vi "Connection Handler.vi"(6 "connection reference":refnum<data-value>, 8 "UUID":string, 9 "Data Model":refnum<class "Device Data Model.lvclass">, 11 "TCP slave":refnum<class "TCP Slave.lvclass">) -> ()   [LabVIEW 2021, in "TCP Slave.lvclass"]
doc: "Handles new connections by waiting on TCP requests. When data is received, it will execute the modbus data unit and write the return data back onto the bus. It handles one request at a time."
uses:
  TCP Slave.lvclass
  TCP Slave.lvclass/TCP Slave.ctl
  Handler State.ctl
  Transmission Data Unit/Transmission Data Unit.lvclass
  Data Model/Device Data Model.lvclass
  Network Slave.lvclass
  C:/my_projects/projects/Algorithms/Labview/21/Modbus_v121c/Network Protocol/Network Slave/Network Slave.lvclass
  C:/my_projects/projects/Algorithms/Labview/21/Modbus_v121c/Network Protocol/Network Protocol.lvclass
  C:/my_projects/projects/Algorithms/Labview/21/Modbus_v121c/Network Protocol/Network Slave/TCP/TCP Slave.lvclass
  Connection.ctl
panel:
  in  "stop":bool
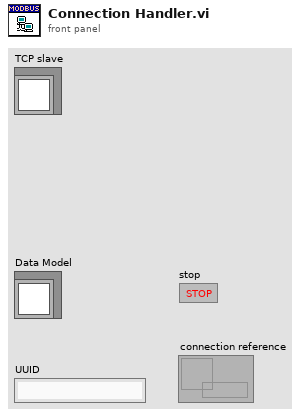
[diagram p1: front panel]
types:
  T1 = typedef "TCP Slave.lvclass/Handler State.ctl" = enum16{"Check Notifier", "Wait on Connection", "Quit"}
  T2 = typedef "TCP Slave.lvclass/Connection.ctl" = cluster{"Connected?":bool, "IP address":string, "connection error":errorcluster}
  T3 = typedef "TCP Slave.lvclass/Connection Counter.ctl" = cluster{"Currently Connected":u32, "Connection Records":refnum<data-value>[]}
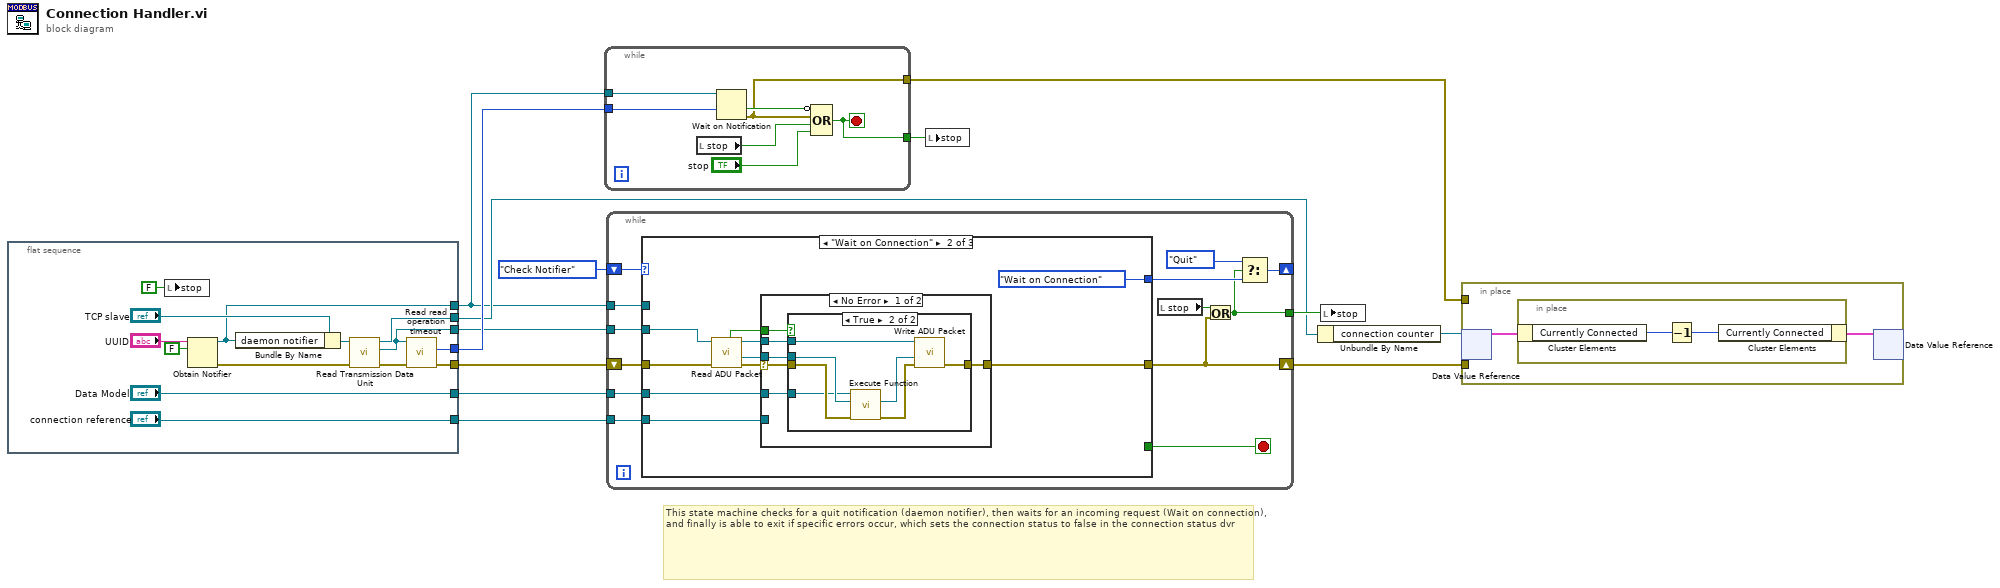
[diagram p0: block diagram]
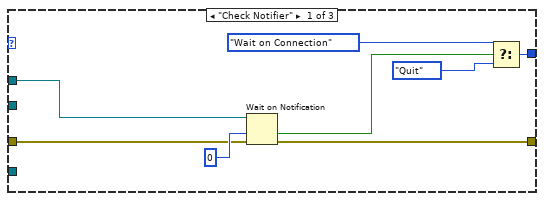
[diagram p2: hidden frame]
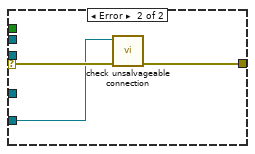
[diagram p4: hidden frame]
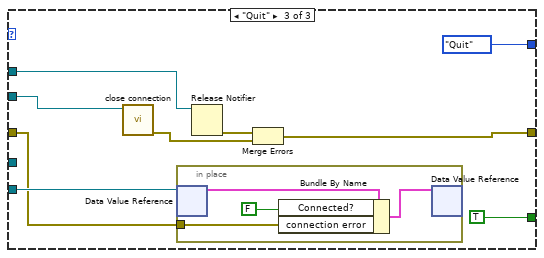
[diagram p5: hidden frame]
diagram:
  # "This state machine checks for a quit notification (daemon notifier), then waits for an incoming request (Wait on connection), and finally is able to exit if specific errors occur, which sets the connection status to false in the connection status dvr"
  n1 = flat-sequence {
    tunnel: ["connection reference"] -> w12
    tunnel: ["Data Model"] -> w11
    tunnel: [w20] -> w6
    tunnel: [w19] -> w5
    tunnel: [w17] -> w4
    tunnel: [w16] -> w1
    tunnel: [w14] -> w3
    frame #0 {
      n2 = local write "stop"(FALSE ("stop")) -> ()
      n3 = Obtain Notifier(name (unnamed)="UUID", notification data type=FALSE) -> (notifier out=w16:refnum<notifier>, error out=w21:errorcluster)  [unwired: 2 in, 1 out]
      n4 = Bundle By Name(cluster="TCP slave", "daemon notifier"=w16) -> (w18:refnum<class "TCP Slave.lvclass">)
      n5 = call "Read Transmission Data Unit.vi"("error in (no error)"=w21, "Network Slave in"=w18) -> ("error out"=w22:errorcluster, "Transmission Data Unit"=w14:refnum<class "Transmission Data Unit.lvclass">, "Network Slave out"=w17:refnum<class "TCP Slave.lvclass">)  [unwired: 7 in]
      n6 = call "Read read operation timeout.vi"("error in (no error)"=w22, "transmission data unit in"=w14) -> ("error out"=w20:errorcluster, "read operation timeout"=w19:i32)  [unwired: 7 in, 1 out]
    }
  }
  n7 = while {
    tunnel: w1 -> [w34]
    tunnel: [w31] -> w8
    tunnel: [w30] -> w2
    tunnel: w5 -> [w28]
    stop <- w31 stop-if-true
    n8 = local read "stop"() -> (w32:bool)
    n9 = Wait on Notification(notifier=w34, timeout in ms (-1)=w28) -> (timed out?=w33:bool, error out=w30:errorcluster)  [unwired: 2 in, 2 out]
    n10 = Compound Arithmetic op=OR(invert w33, w30, w32, "stop") -> (w31:bool)
  }
  n11 = while {
    shift-right: [w45] -> _
    shift-left: Handler_State."Check Notifier" ("Listener State") -> [w47]
    shift-right: [w37] -> w10
    shift-left: w6 -> [w42]
    tunnel: w12 -> [w40]
    tunnel: w11 -> [w39]
    tunnel: [w36] -> w7
    tunnel: w1 -> [w41]
    tunnel: w3 -> [w35]
    stop <- w43 stop-if-true
    n12 = case shown="\"Wait on Connection\"" w47 {
      tunnel: [w49 Handler_State."Wait on Connection" ("Listener State") Handler_State."Quit" ("Listener State")] -> w44
      tunnel: [_ _ TRUE] -> w43
      tunnel: [w54 w61 w88] -> w37
      tunnel: w42 -> [w53 w56 w85]
      tunnel: w41 -> [w48 _ w86]
      tunnel: w40 -> [_ w60 w89]
      tunnel: w39 -> [_ w59 _]
      tunnel: w35 -> [_ w57 w83]
      frame "Check Notifier" {
        n13 = Wait on Notification(notifier=w48, timeout in ms (-1)=0, error in (no error)=w53) -> (timed out?=w52:bool, error out=w54:errorcluster)  [unwired: 1 in, 2 out]
        n14 = Select(t=Handler_State."Wait on Connection" ("Listener State"), s=w52, f=Handler_State."Quit" ("Listener State")) -> (s? t:f=w49:T1)
      }
      frame "Wait on Connection" {
        n15 = call-dynamic "Read ADU Packet.vi"("error in"=w56, "transmission data unit in"=w57) -> ("error out"=w64:errorcluster, "modbus data unit"=w62:refnum<class "Modbus Data Unit.lvclass">, "transmission data unit out"=w63:refnum<class "Transmission Data Unit.lvclass">, "PDU Valid?"=w58:bool)  [unwired: 6 in]
        n16 = case shown="No Error" w64 {
          selector: w64 -> [w68 w82]
          tunnel: w63 -> [w71 _]
          tunnel: w62 -> [w70 _]
          tunnel: [w69 w81] -> w61
          tunnel: w60 -> [_ w80]
          tunnel: w59 -> [w67 _]
          tunnel: w58 -> [w66 _]
          frame No Error {
            n17 = case shown="True" w66 {
              tunnel: w71 -> [_ w79]
              tunnel: w70 -> [_ w78]
              tunnel: [w72 w76] -> w69
              tunnel: w68 -> [w72 w75]
              tunnel: w67 -> [_ w73]
              frame False {
              }
              frame True {
                n18 = call-dynamic "Execute Function.vi"("error in"=w75, "modbus request"=w78, "device data model in"=w73) -> ("error out"=w74:errorcluster, "modbus response"=w77:refnum<class "Modbus Data Unit.lvclass">)  [unwired: 6 in, 1 out]
                n19 = call-dynamic "Write ADU Packet.vi"("error in"=w74, "modbus data unit"=w77, "transmission data unit in"=w79) -> ("error out"=w76:errorcluster)  [unwired: 7 in, 1 out]
              }
            }
          }
          frame Error {
            n20 = call "check unsalvageable connection.vi"("error in (no error)"=w82, "connection reference"=w80) -> ("error out"=w81:errorcluster)  [unwired: 9 in]
          }
        }
      }
      frame "Quit" {
        n21 = call-dynamic "close connection.vi"("transmission data unit in"=w83) -> ("error out"=w84:errorcluster)  [unwired: 9 in, 1 out]
        n22 = in-place {
          in-place-border: w85 -> [w92]
          n23 = in-place-dvr #1(w89) -> (w95:T2)  [unwired: 1 out]
          n24 = Bundle By Name(cluster=w95, "Connected?"=FALSE, "connection error"=w92) -> (w93:T2)
          n25 = in-place-dvr #1(w93) -> ()  [unwired: 2 out]
        }
        n26 = Release Notifier(notifier=w86) -> (error out=w87:errorcluster)  [unwired: 2 in, 2 out]
        n27 = Merge Errors(w87, w84) -> (w88:errorcluster)
      }
    }
    n28 = local read "stop"() -> (w38:bool)
    n29 = Or(x=w38, y=w37) -> (x .or. y?=w36:bool)
    n30 = Select(t=Handler_State."Quit" ("Listener State"), s=w36, f=w44) -> (s? t:f=w45:T1)
  }
  n31 = local write "stop"(w8) -> ()
  n32 = Unbundle By Name(w4) -> ("connection counter"=w9:refnum<data-value>)
  n33 = local write "stop"(w7) -> ()
  n34 = in-place {
    in-place-border: w10 -> [_]
    in-place-border: w2 -> [_]
    n35 = in-place-dvr #2(w9) -> (w97:T3)  [unwired: 1 out]
    n36 = in-place {
      n37 = in-place-cluster #3(w97) -> ("Currently Connected"=w99:u32)
      n38 = Decrement(x=w99) -> (x-1=w98:u32)
      n39 = in-place-cluster #3("Currently Connected"=w98) -> (w96:T3)
    }
    n40 = in-place-dvr #2(w96) -> ()  [unwired: 2 out]
  }
